vi "Close Listener.vi"(8 "error in (no error)":errorcluster, 11 "TCP slave in":refnum<class "TCP Slave.lvclass">) -> (0 "error out":errorcluster, 3 "TCP slave out":refnum<class "TCP Slave.lvclass">)   [LabVIEW 2015, in "SubVIs.lvlib" / "TCP Slave.lvclass"]
doc: "Closes the TCP listener."
uses:
  <vilib>/Modbus/subvis/Protocol/TCP/TCP Slave/TCP Slave.lvclass
  <vilib>/Modbus/subvis/Protocol/TCP/TCP Slave/TCP Slave.lvclass/TCP Slave.ctl
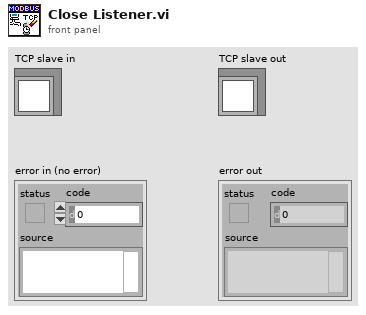
[diagram p1: front panel]
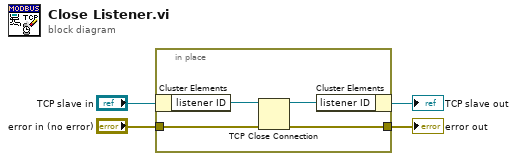
[diagram p0: block diagram]
diagram:
  n1 = in-place {
    in-place-border: "error in (no error)" -> [w8]
    in-place-border: [w7] -> w3
    n2 = in-place-cluster #1("TCP slave in") -> ("listener ID"=w5:refnum<k5>)
    n3 = TCP Close Connection(connection ID=w5, error in (no error)=w8) -> (connection ID out=w6:refnum<k5>, error out=w7:errorcluster)  [unwired: 1 in]
    n4 = in-place-cluster #1("listener ID"=w6) -> (→"TCP slave out":refnum<class "TCP Slave.lvclass">)
  }
  "error out" <- w3
